vi "交换探头地址.vi"(8 "引用输入":T1, 11 "点到行列-实时列表":T2 caption="行和列") -> (2 "回滚成功？":bool, 3 "设置成功？":bool)   [LabVIEW 2017]
uses:
  <vilib>/Utility/miscctls.llb/LVRowAndColumnTypeDef.ctl
panel:
  out "引用-暂停发送":refnum<vi>
  in  "取消":bool
  in  "确定":bool
  in  "交换到探头":u8=1 min=1 max=35
  out "被修改探头":u8
  # "交换探头地址"
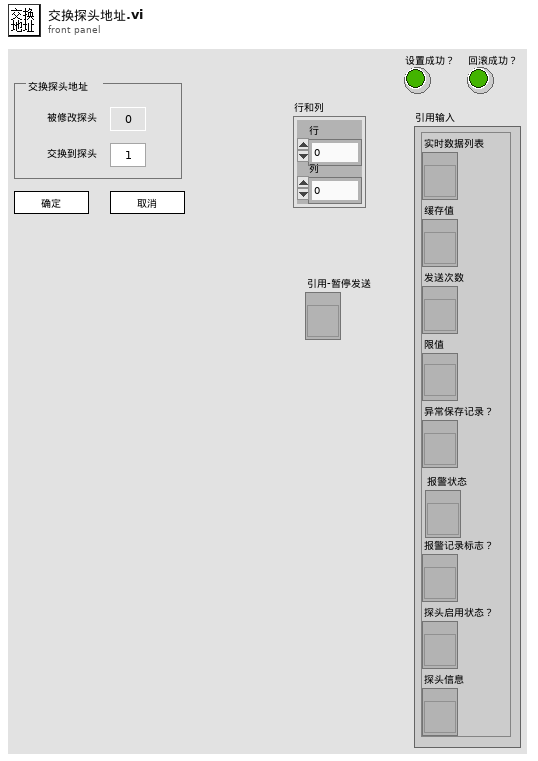
[diagram p1: front panel]
types:
  T1 = cluster{"实时数据列表":refnum<vi>, "缓存值":refnum<vi>, "发送次数":refnum<vi>, "限值":refnum<vi>, "异常保存记录？":refnum<vi>, "报警记录标志？":refnum<vi>, "探头启用状态？":refnum<vi>, "探头信息":refnum<vi>, "报警状态":refnum<vi>}
  T2 = typedef "LVRowAndColumnTypeDef.ctl" = cluster{"Row":i32, "Column":i32}
  T3 = enum32{"Invalid", "Standard", "Closed", "Hidden", "Minimized", "Maximized"}
  T4 = cluster{"限值1":dbl, "限值2":dbl, "探头限值":enum16{"一级限值", "二级限值"}}[]
  T5 = cluster{"限值1":dbl, "限值2":dbl, "探头限值":enum16{"一级限值", "二级限值"}}
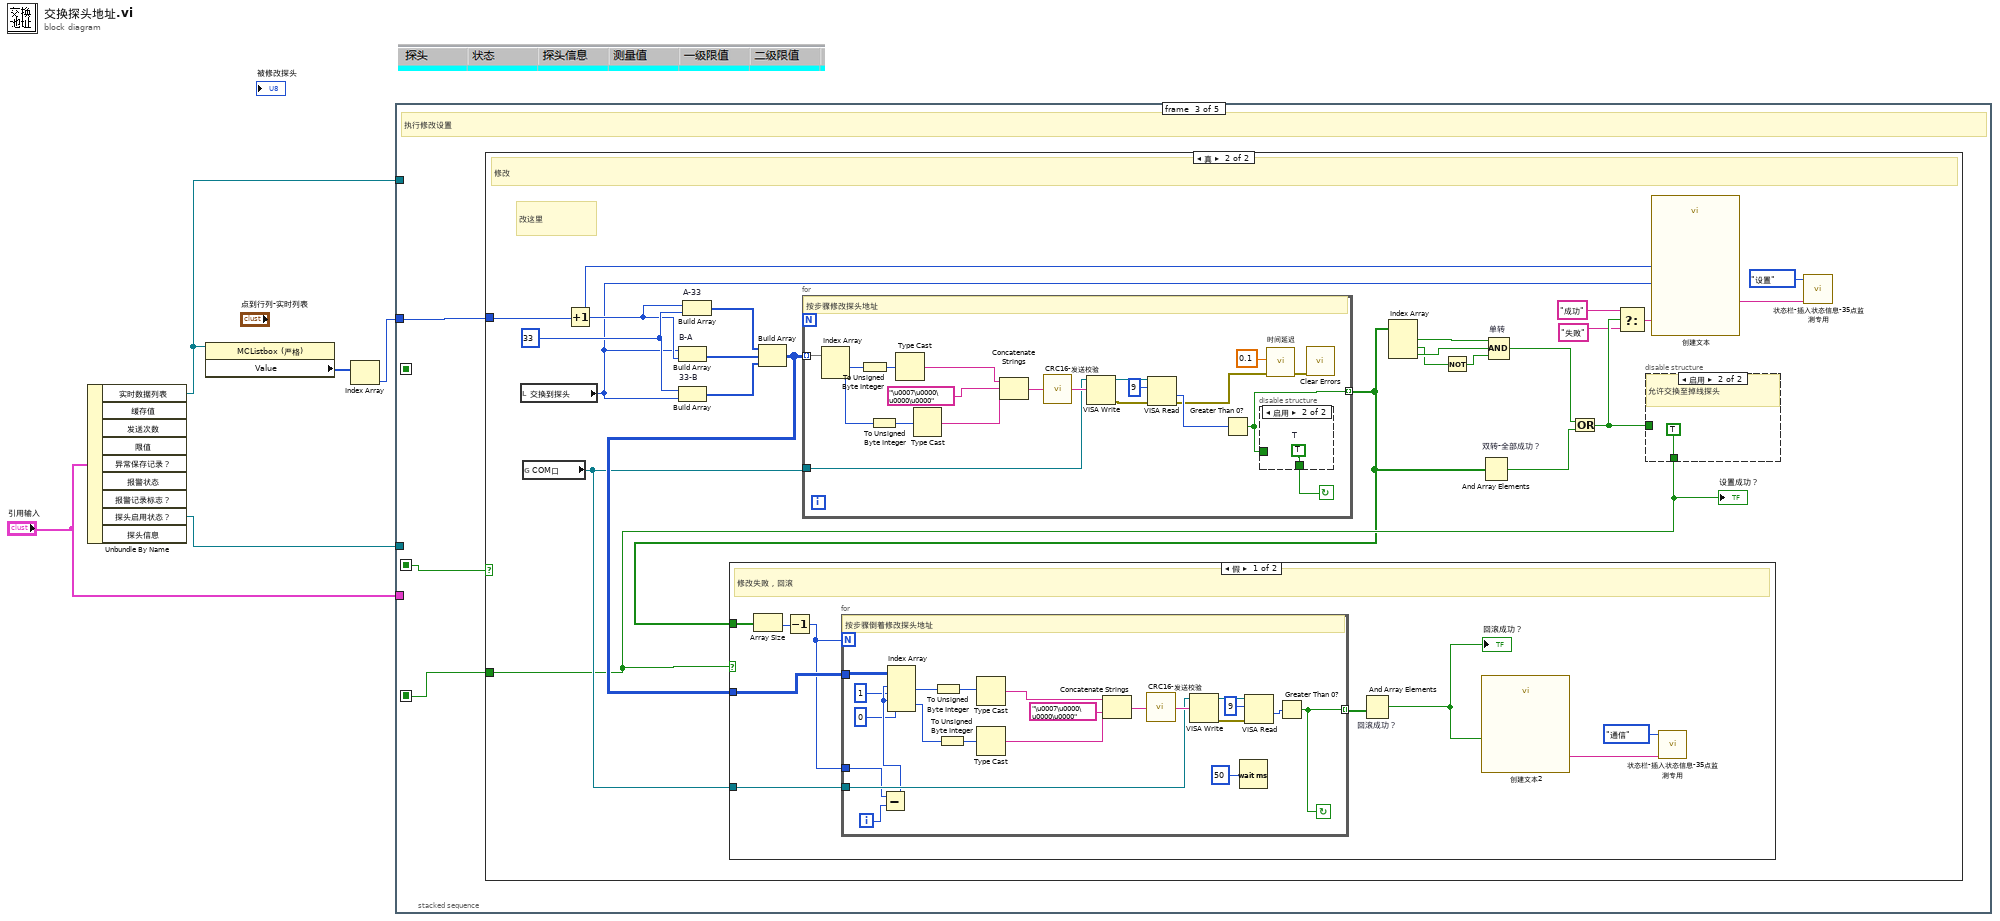
[diagram p0: block diagram]
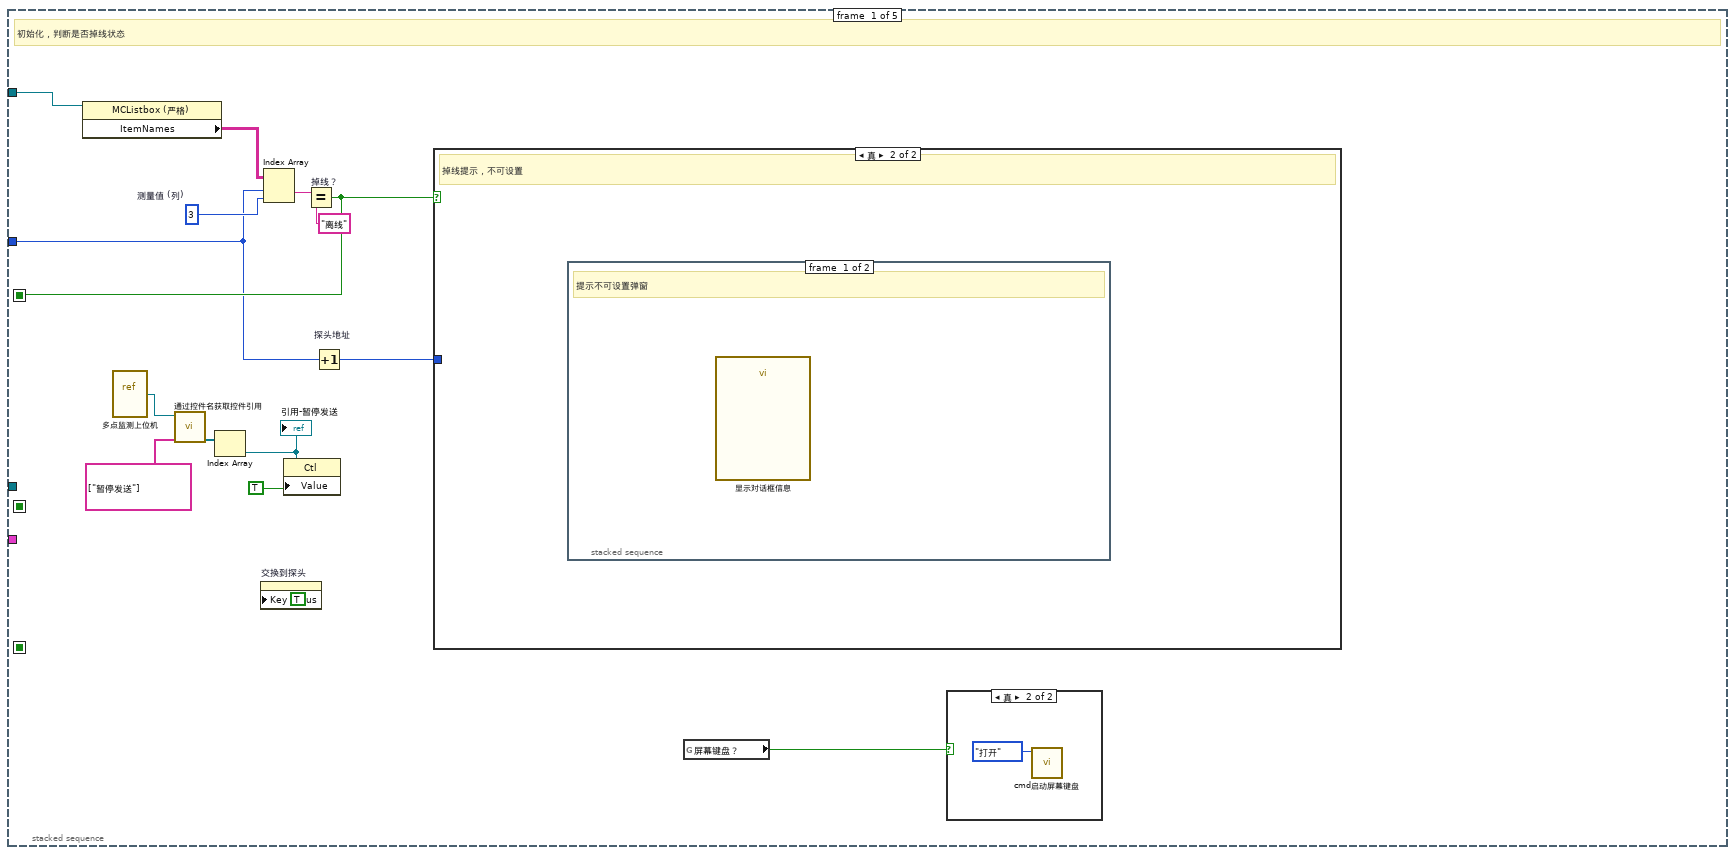
[diagram p2: hidden frame]
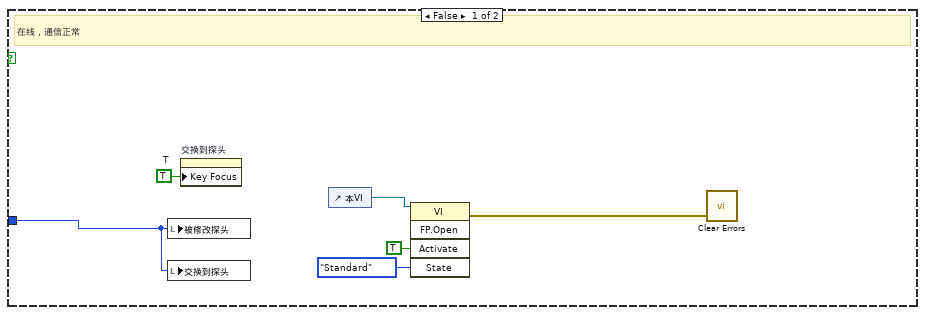
[diagram p4: hidden frame]
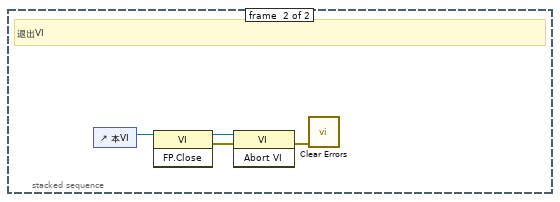
[diagram p5: hidden frame]
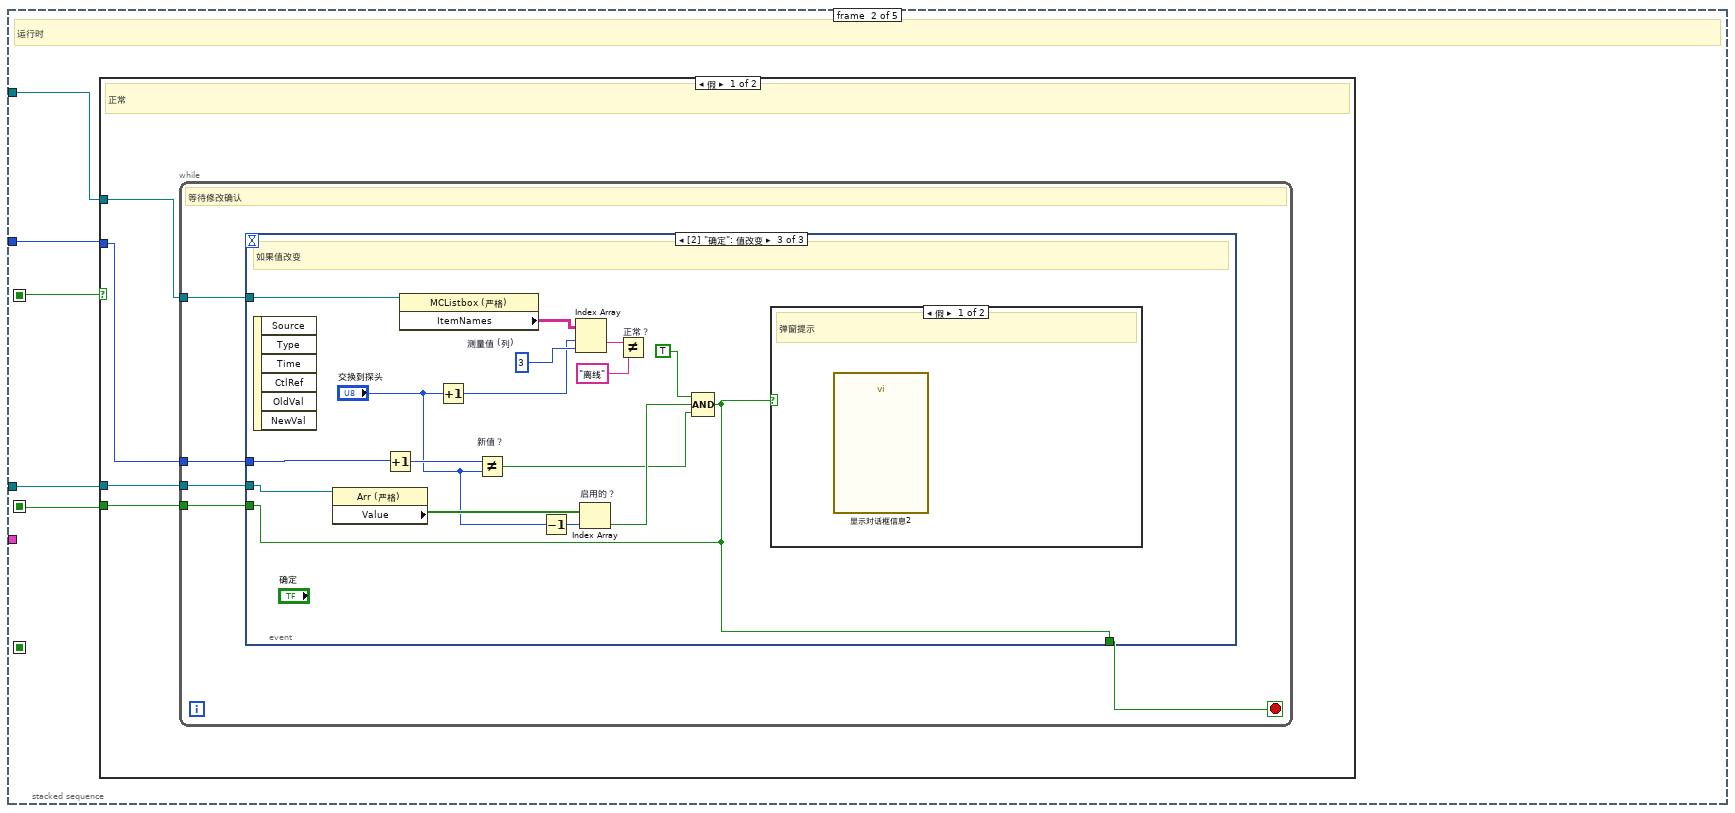
[diagram p6: hidden frame]
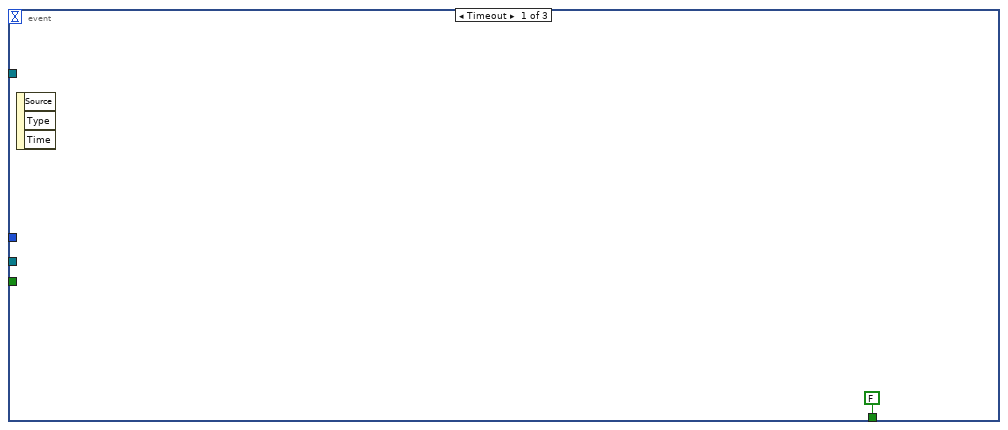
[diagram p7: hidden frame]
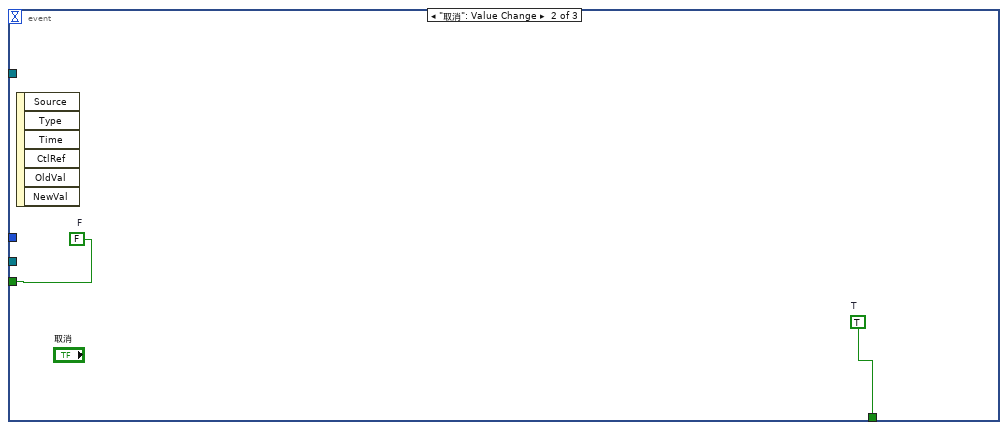
[diagram p8: hidden frame]
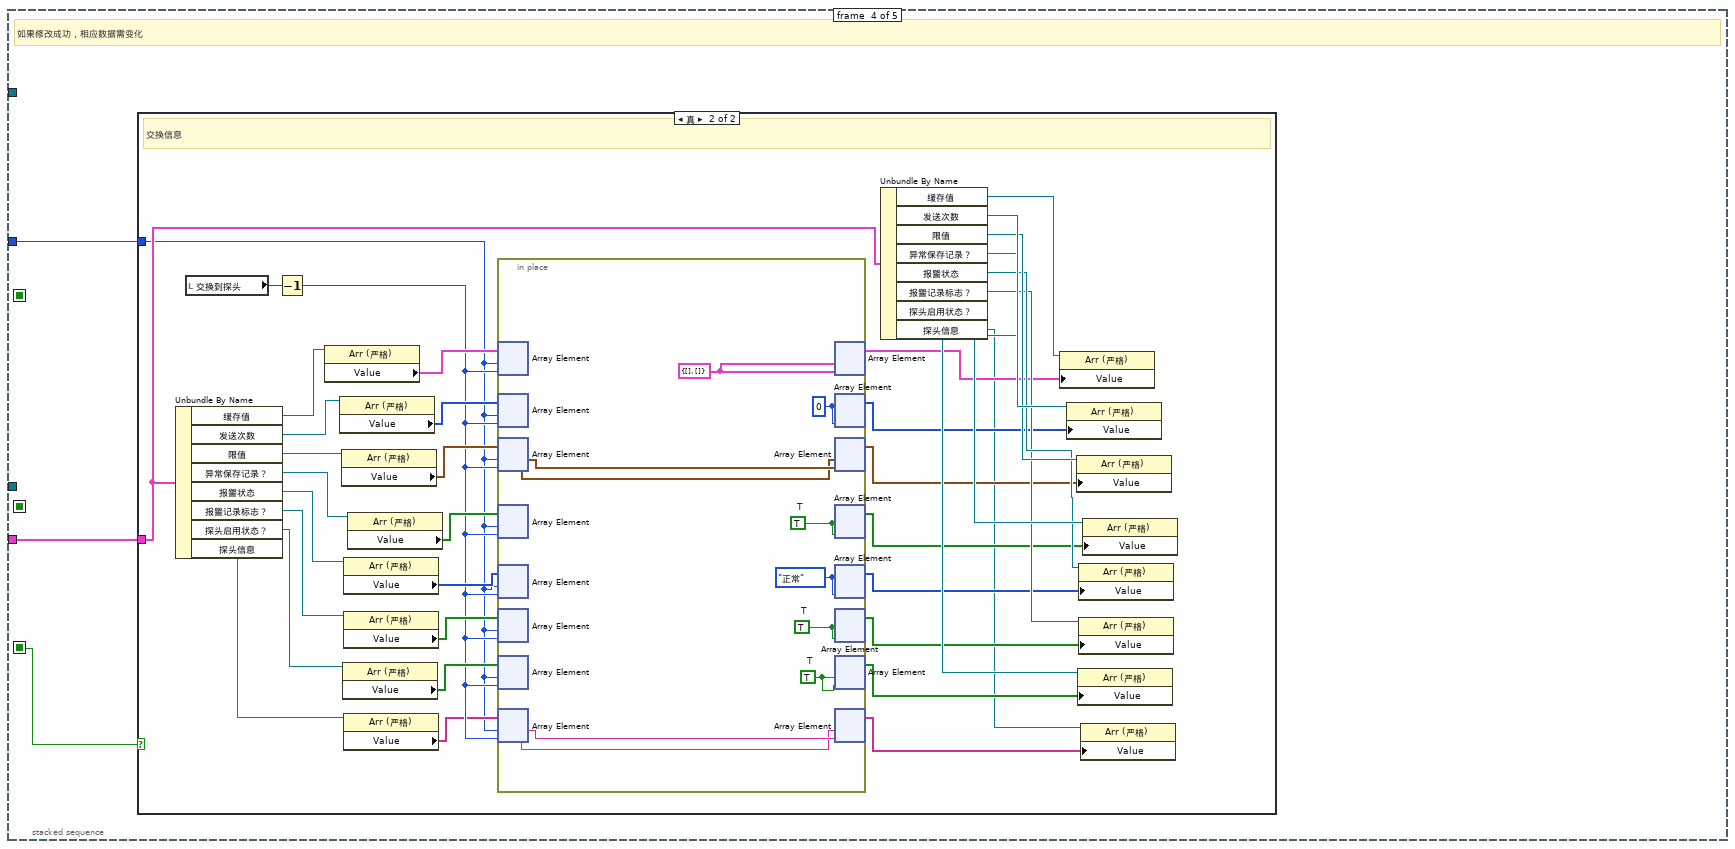
[diagram p15: hidden frame]
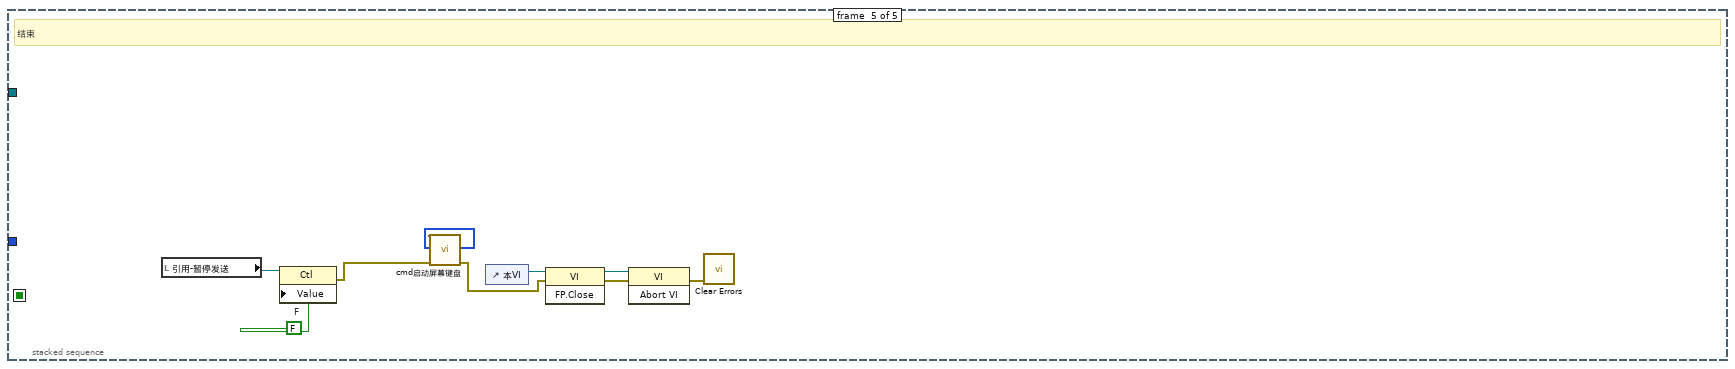
[diagram p17: hidden frame]
diagram:
  n1 = Unbundle By Name("引用输入") -> ("实时数据列表"=w3:refnum<vi>, "探头启用状态？"=w5:refnum<vi>)  [unwired: 7 out]
  n2 = property class="MCListbox (严格)"(reference=w3) -> ("Value"=w2:i32[])  [unwired: 1 in, 2 out]
  n3 = Index Array(array=w2) -> (element=w1:i32)  [unwired: 1 in]
  n4 = stacked-sequence {
    seq-local: [w15 _ _ _ _] -> [_ w36 _ _ _]
    seq-local: [_ w35 _ _ _] -> [_ _ w67 _ _]
    seq-local: [_ _ w66 _ _] -> [_ _ _ w148 _]
    tunnel: w3 -> [w20 w34 _ _ _]
    tunnel: w5 -> [_ w33 _ _ _]
    tunnel: "引用输入" -> [_ _ _ w147 _]
    tunnel: w1 -> [w13 w32 w65 w146 _]
    frame #0 {
      w18 = 3  # 测量值 (列)
      # "初始化，判断是否掉线状态"
      n5 = property class="MCListbox (严格)"(reference=w20) -> ("ItemNames"=w19:string[][])  [unwired: 1 in, 2 out]
      n6 = vi-ref "多点监测上位机.vi"() -> (w8:refnum<vi>)
      n7 = call "通过控件名获取控件引用.vi"("控件名数组"=string[] ["暂停发送"], "VI引用"=w8) -> ("控件引用输出"=w11:refnum<vi>[])  [unwired: 7 in, 2 out]
      n8 = Index Array(array=w11) -> (element=w9:refnum<vi>)  [unwired: 1 in]
      "引用-暂停发送" <- w9
      n9 = property on="交换到探头" class="DigNum (严格)"("Key Focus"=TRUE ("键选中")) -> ()  [unwired: 2 in, 2 out]
      n10 = Index Array(array=w19, index (row)=w13, index (col)=w18) -> (element=w17:string)
      n11 = property class="Ctl"(reference=w9, "Value"=TRUE ("T")) -> ()  [unwired: 1 in, 2 out]
      n12 = Equal? "掉线？"(x=w17, y="离线") -> (x = y?=w15:bool)
      n13 = Increment "探头地址"(x=w13) -> (x+1=w14:i32)
      n14 = case shown="真" w15 {
        tunnel: w14 -> [w27 _]
        frame False {
          w26 = TRUE  # T
          # "在线，通信正常"
          n15 = local write "被修改探头"(w27) -> ()
          n16 = local write "交换到探头"(w27) -> ()
          n17 = property on="交换到探头" class="DigNum (严格)"("Key Focus"=w26) -> ()  [unwired: 2 in, 2 out]
          n18 = control-ref of="本VI"() -> (w25:refnum<vi>)
          n19 = invoke class="VI" method="FP.Open"(reference=w25, "Activate"=TRUE ("激活？"), "State"=T3."Standard" ("状态")) -> (error out=w22:errorcluster)  [unwired: 2 in, 4 out]
          n20 = call <vilib>:"Clear Errors.vi"("error in (no error)"=w22) -> ()  [unwired: 5 in, 2 out]
        }
        frame True {
          # "掉线提示，不可设置"
          n21 = stacked-sequence {
            frame #0 {
              # "提示不可设置弹窗"
              n22 = call "显示对话框信息"() -> ()  [unwired: 10 in, 2 out]
            }
            frame #1 {
              # "退出VI"
              n23 = control-ref of="本VI"() -> (w31:refnum<vi>)
              n24 = invoke class="VI" method="FP.Close"(reference=w31) -> (reference out=w30:refnum<vi>, error out=w29:errorcluster)  [unwired: 2 in, 1 out]
              n25 = invoke class="VI" method="Abort VI"(reference=w30, error in=w29) -> (error out=w28:errorcluster)  [unwired: 1 in, 2 out]
              n26 = call <vilib>:"Clear Errors.vi"("error in (no error)"=w28) -> ()  [unwired: 5 in, 2 out]
            }
          }
        }
      }
      n27 = global read "全局变量-35点监测.vi" "屏幕键盘？"() -> (w6:bool)
      n28 = case shown="真" w6 {
        frame False {
        }
        frame True {
          n29 = call "cmd启动屏幕键盘.vi"("软键盘开关"=enum16{"关闭", "打开"}."打开") -> ()  [unwired: 9 in, 2 out]
        }
      }
    }
    frame #1 {
      # "运行时"
      n30 = case shown="假" w36 {
        tunnel: w32 -> [w39 _]
        tunnel: [w40 _] -> w35
        tunnel: w34 -> [w38 _]
        tunnel: w33 -> [w37 _]
        frame False {
          # "正常"
          n31 = while {
            tunnel: [w44] -> w40
            tunnel: w39 -> [w43]
            tunnel: w38 -> [w42]
            tunnel: w37 -> [w41]
            stop <- w45 stop-if-true
            # "等待修改确认"
            n32 = event shown="[2] \"确定\": 值改变" {
              selector: _ -> [_ _ _]
              dyn-events: _ -> [_ _ _]
              timeout: _ -> [_ _ _]
              tunnel: [FALSE ("T") w48 w54] -> w45
              tunnel: [_ w47 w54] -> w44
              tunnel: w43 -> [_ _ w53]
              tunnel: w42 -> [_ _ w59]
              tunnel: w41 -> [_ _ w58]
              event Timeout {
                n33 = event-data() -> ()  [unwired: 1 in, 3 out]
              }
              event "取消": Value Change {
                w47 = FALSE  # F
                w48 = TRUE  # T
                n34 = event-data() -> ()  [unwired: 1 in, 6 out]
              }
              event "确定": Value Change {
                w62 = 3  # 测量值 (列)
                # "如果值改变"
                n35 = event-data() -> ()  [unwired: 1 in, 6 out]
                n36 = property class="Arr (严格)"(reference=w58) -> ("Value"=w57:bool[])  [unwired: 1 in, 2 out]
                n37 = Increment(x=w53) -> (x+1=w64:i32)
                n38 = property class="MCListbox (严格)"(reference=w59) -> ("ItemNames"=w63:string[][])  [unwired: 1 in, 2 out]
                n39 = Increment(x="交换到探头") -> (x+1=w51:u8)
                n40 = Not Equal? "新值？"(x=w64, y="交换到探头") -> (x != y?=w55:bool)
                n41 = Decrement(x="交换到探头") -> (x-1=w49:u8)
                n42 = Index Array(array=w63, index (row)=w51, index (col)=w62) -> (element=w61:string)
                n43 = Index Array "启用的？"(array=w57, index=w49) -> (element=w56:bool)
                n44 = Not Equal? "正常？"(x=w61, y="离线") -> ()  [unwired: 1 out]
                n45 = Compound Arithmetic op=AND(TRUE ("值"), w56, w55) -> (w54:bool)
                n46 = case shown="假" w54 {
                  frame False {
                    # "弹窗提示"
                    n47 = call "显示对话框信息2"() -> ()  [unwired: 10 in, 2 out]
                  }
                  frame True {
                    # "正常，启用，新值"
                  }
                }
              }
            }
          }
        }
        frame True {
          # "掉线"
        }
      }
    }
    frame #2 {
      # "执行修改设置"
      n48 = case shown="真" w67 {
        tunnel: [_ w78] -> w66
        tunnel: w65 -> [_ w79]
        frame False {
          # "不执行"
        }
        frame True {
          w90 = 33 ("元素")
          # "改这里"
          # "修改"
          n49 = local read "交换到探头"() -> (w81:u8)
          n50 = global read "全局变量-35点监测.vi" "COM口"() -> (w84:refnum<visa-resource-name>)
          n51 = Increment(x=w79) -> (x+1=w82:i32)
          n52 = Build Array "B-A"(w81, w82) -> (w88:i32[])
          n53 = Build Array "33-B"(w90, w81) -> (w87:i32[])
          n54 = Build Array "A-33"(w82, w90) -> (w89:i32[])
          n55 = Build Array(w89, w88, w87) -> (w85:i32[][])
          n56 = for {
            tunnel: w85 -> [w143] mode=indexing
            tunnel: w84 -> [w131]
            tunnel: [w128] -> w73 mode=indexing
            stop <- w129 continue-if-true
            # "按步骤修改探头地址"
            n57 = Index Array(array=w143) -> (element #1=w137:i32, element #2=w136:i32)  [unwired: 2 in]
            n58 = To Unsigned Byte Integer(number=w137) -> (unsigned 8bit integer=w142:u8)
            n59 = To Unsigned Byte Integer(number=w136) -> (unsigned 8bit integer=w141:u8)
            n60 = Type Cast(x=w142) -> (*(type *) &x=w139:string)  [unwired: 1 in]
            n61 = Type Cast(x=w141) -> (*(type *) &x=w138:string)  [unwired: 1 in]
            n62 = Concatenate Strings(w139, "\u0007\u0000\u0000\u0000", w138) -> (w135:string)
            n63 = call "CRC16-发送校验.vi"("净数据"=w135) -> ("完整输出"=w132:string)
            n64 = VISA Write(VISA resource name=w131, write buffer=w132) -> (VISA resource name out=w134:refnum<visa-resource-name>, error out=w124:errorcluster)  [unwired: 1 in, 1 out]
            n65 = VISA Read(VISA resource name=w134, byte count=u32 9 ("字节总数"), error in (no error)=w124) -> (return count=w130:u32, error out=w127:errorcluster)  [unwired: 2 out]
            n66 = Greater Than 0?(x=w130) -> (x > 0?=w128:bool)
            n67 = disable-structure shown="启用" {
              disable-tunnel: [w144 w145] -> w129
              disable-tunnel: w128 -> [w144 _]
              frame Disabled {
              }
              frame Enabled {
                w145 = TRUE  # T
              }
            }
            n68 = call "时间延迟"("error in (no error)"=w127, "Delay Time (s)"=0.1) -> ("error out"=w126:errorcluster)  [unwired: 9 in]
            n69 = call <vilib>:"Clear Errors.vi"("error in (no error)"=w126) -> ()  [unwired: 5 in, 2 out]
          }
          n70 = Index Array(array=w73) -> (element #1=w72:bool, element #2=w70:bool, element #3=w71:bool)  [unwired: 3 in]
          n71 = Not(x=w70) -> (.not. x?=w69:bool)
          n72 = And Array Elements "双转-全部成功？"(Boolean array=w73) -> (logical AND=w86:bool)
          n73 = Compound Arithmetic op=AND "单转"(w72, w71, w69) -> (w68:bool)
          n74 = Or(x=w68, y=w86) -> (x .or. y?=w77:bool)
          n75 = Select(t="成功", s=w77, f="失败") -> (s? t:f=w74:string)
          n76 = disable-structure shown="启用" {
            disable-tunnel: w77 -> [w91 _]
            disable-tunnel: [w91 TRUE ("设置成功？")] -> w78
            frame Disabled {
              # "不允许交换至掉线探头"
            }
            frame Enabled {
              # "允许交换至掉线探头"
            }
          }
          "设置成功？" <- w78
          n77 = case shown="假" w78 {
            tunnel: w73 -> [w101 _]
            tunnel: w85 -> [w99 _]
            tunnel: w84 -> [w98 _]
            frame False {
              # "修改失败，回滚"
              n78 = Array Size(array=w101) -> (size(s)=w100:i32)
              n79 = Decrement(x=w100) -> (x-1=w97:i32)
              n80 = for {
                N: w97 -> [_]
                tunnel: w99 -> [w123]
                tunnel: w98 -> [w110]
                tunnel: [w107] -> w96 mode=indexing
                tunnel: w97 -> [w105]
                i -> [w106]
                stop <- w107 continue-if-true
                # "按步骤倒着修改探头地址"
                n81 = Subtract(x=w105, y=w106) -> (x-y=w104:i32)
                n82 = Index Array(array=w123, index (row) #1=w104, index (col) #1=1 ("禁用的索引 (列)"), index (row) #2=w104, index (col) #2=0 ("禁用的索引 (列)")) -> (element #1=w117:i32, element #2=w116:i32)
                n83 = To Unsigned Byte Integer(number=w117) -> (unsigned 8bit integer=w122:u8)
                n84 = To Unsigned Byte Integer(number=w116) -> (unsigned 8bit integer=w121:u8)
                n85 = Type Cast(x=w122) -> (*(type *) &x=w119:string)  [unwired: 1 in]
                n86 = Type Cast(x=w121) -> (*(type *) &x=w118:string)  [unwired: 1 in]
                n87 = Concatenate Strings(w119, "\u0007\u0000\u0000\u0000", w118) -> (w115:string)
                n88 = call "CRC16-发送校验.vi"("净数据"=w115) -> ("完整输出"=w111:string)
                n89 = VISA Write(VISA resource name=w110, write buffer=w111) -> (VISA resource name out=w113:refnum<visa-resource-name>, error out=w114:errorcluster)  [unwired: 1 in, 1 out]
                n90 = Wait (ms)(milliseconds to wait=u32 50 ("等待时间（毫秒）")) -> ()  [unwired: 1 out]
                n91 = VISA Read(VISA resource name=w113, byte count=u32 9 ("字节总数"), error in (no error)=w114) -> (return count=w108:u32)  [unwired: 3 out]
                n92 = Greater Than 0?(x=w108) -> (x > 0?=w107:bool)
              }
              n93 = And Array Elements "回滚成功？"(Boolean array=w96) -> (logical AND=w94:bool)
              "回滚成功？" <- w94
              n94 = call "创建文本2"("回滚成功？"=w94) -> ("Result"=w93:string)  [unwired: 13 in, 1 out]
              n95 = call "状态栏-插入状态信息-35点监测专用.vi"("消息内容"=w93, "状态类型"=enum16{"全部", "报警", "通信", "设置"}."通信") -> ()  [unwired: 10 in]
            }
            frame True {
              # "修改成功"
            }
          }
          n96 = call "创建文本"("从探头"=w82, "到探头"=w81, "交换结果"=w74) -> ("Result"=w80:string)  [unwired: 11 in, 1 out]
          n97 = call "状态栏-插入状态信息-35点监测专用.vi"("消息内容"=w80, "状态类型"=enum16{"全部", "报警", "通信", "设置"}."设置") -> ()  [unwired: 10 in]
        }
      }
    }
    frame #3 {
      # "如果修改成功，相应数据需变化"
      n98 = case shown="真" w148 {
        tunnel: w147 -> [_ w169]
        tunnel: w146 -> [_ w149]
        frame False {
        }
        frame True {
          # "交换信息"
          n99 = Unbundle By Name(w169) -> ("缓存值"=w183:refnum<vi>, "发送次数"=w181:refnum<vi>, "限值"=w179:refnum<vi>, "异常保存记录？"=w177:refnum<vi>, "报警状态"=w175:refnum<vi>, "报警记录标志？"=w173:refnum<vi>, "探头启用状态？"=w172:refnum<vi>, "探头信息"=w154:refnum<vi>)
          n100 = local read "交换到探头"() -> (w184:u8)
          n101 = Decrement(x=w184) -> (x-1=w153:u8)
          n102 = property class="Arr (严格)"(reference=w183) -> ("Value"=w182:cluster{"X":timestamp[], "Y":dbl[]}[])  [unwired: 1 in, 2 out]
          n103 = property class="Arr (严格)"(reference=w181) -> ("Value"=w180:u8[])  [unwired: 1 in, 2 out]
          n104 = property class="Arr (严格)"(reference=w179) -> ("Value"=w178:T4)  [unwired: 1 in, 2 out]
          n105 = property class="Arr (严格)"(reference=w172) -> ("Value"=w170:bool[])  [unwired: 1 in, 2 out]
          n106 = property class="Arr (严格)"(reference=w175) -> ("Value"=w174:enum16{"正常", "一级报警", "二级报警", "累积报警"}[])  [unwired: 1 in, 2 out]
          n107 = property class="Arr (严格)"(reference=w173) -> ("Value"=w171:bool[])  [unwired: 1 in, 2 out]
          n108 = property class="Arr (严格)"(reference=w154) -> ("Value"=w152:string[])  [unwired: 1 in, 2 out]
          n109 = property class="Arr (严格)"(reference=w177) -> ("Value"=w176:bool[])  [unwired: 1 in, 2 out]
          n110 = in-place {
            w187 = TRUE  # T
            w188 = TRUE  # T
            w189 = enum16{"正常", "一级报警", "二级报警"}."正常" ("元素")
            w190 = TRUE  # T
            w193 = u8 0 ("元素")
            w194 = cluster{"X":timestamp[], "Y":dbl[]} {"X"=[], "Y"=[]} ("元素")
            n111 = in-place-array #1(w182, w149, w153) -> ()  [unwired: 2 out]
            n112 = in-place-array #2(w180, w149, w153) -> ()  [unwired: 2 out]
            n113 = in-place-array #3(w178, w149, w153) -> (w192:T5, w191:T5)
            n114 = in-place-array #4(w176, w149, w153) -> ()  [unwired: 2 out]
            n115 = in-place-array #5(w174, w149, w153) -> ()  [unwired: 2 out]
            n116 = in-place-array #6(w171, w149, w153) -> ()  [unwired: 2 out]
            n117 = in-place-array #7(w170, w149, w153) -> ()  [unwired: 2 out]
            n118 = in-place-array #8(w152, w149, w153) -> (w186:string, w185:string)
            n119 = in-place-array #1(w194, w194) -> (w161:cluster{"X":timestamp[], "Y":dbl[]}[])  [unwired: 2 out]
            n120 = in-place-array #2(w193, w193) -> (w160:u8[])  [unwired: 2 out]
            n121 = in-place-array #3(w191, w192) -> (w159:T4)  [unwired: 2 out]
            n122 = in-place-array #4(w190, w190) -> (w158:bool[])  [unwired: 2 out]
            n123 = in-place-array #5(w189, w189) -> (w157:enum16{"正常", "一级报警", "二级报警", "累积报警"}[])  [unwired: 2 out]
            n124 = in-place-array #6(w188, w188) -> (w156:bool[])  [unwired: 2 out]
            n125 = in-place-array #7(w187, w187) -> (w155:bool[])  [unwired: 2 out]
            n126 = in-place-array #8(w185, w186) -> (w150:string[])  [unwired: 2 out]
          }
          n127 = Unbundle By Name(w169) -> ("缓存值"=w168:refnum<vi>, "发送次数"=w167:refnum<vi>, "限值"=w166:refnum<vi>, "异常保存记录？"=w165:refnum<vi>, "报警状态"=w164:refnum<vi>, "报警记录标志？"=w163:refnum<vi>, "探头启用状态？"=w162:refnum<vi>, "探头信息"=w151:refnum<vi>)
          n128 = property class="Arr (严格)"(reference=w168, "Value"=w161) -> ()  [unwired: 1 in, 2 out]
          n129 = property class="Arr (严格)"(reference=w167, "Value"=w160) -> ()  [unwired: 1 in, 2 out]
          n130 = property class="Arr (严格)"(reference=w166, "Value"=w159) -> ()  [unwired: 1 in, 2 out]
          n131 = property class="Arr (严格)"(reference=w162, "Value"=w155) -> ()  [unwired: 1 in, 2 out]
          n132 = property class="Arr (严格)"(reference=w164, "Value"=w157) -> ()  [unwired: 1 in, 2 out]
          n133 = property class="Arr (严格)"(reference=w163, "Value"=w156) -> ()  [unwired: 1 in, 2 out]
          n134 = property class="Arr (严格)"(reference=w151, "Value"=w150) -> ()  [unwired: 1 in, 2 out]
          n135 = property class="Arr (严格)"(reference=w165, "Value"=w158) -> ()  [unwired: 1 in, 2 out]
        }
      }
    }
    frame #4 {
      w199 = FALSE  # F
      # "结束"
      n136 = local read "引用-暂停发送"() -> (w198:refnum<vi>)
      n137 = property class="Ctl"(reference=w198, "Value"=w199) -> (error out=w196:errorcluster)  [unwired: 1 in, 1 out]
      n138 = call "cmd启动屏幕键盘.vi"("error in (no error)"=w196, "软键盘开关"=enum16{"关闭", "打开"}."关闭") -> ("error out"=w195:errorcluster)  [unwired: 8 in, 1 out]
      n139 = control-ref of="本VI"() -> (w203:refnum<vi>)
      n140 = invoke class="VI" method="FP.Close"(reference=w203, error in=w195) -> (reference out=w202:refnum<vi>, error out=w201:errorcluster)  [unwired: 1 in, 1 out]
      n141 = invoke class="VI" method="Abort VI"(reference=w202, error in=w201) -> (error out=w200:errorcluster)  [unwired: 1 in, 2 out]
      n142 = call <vilib>:"Clear Errors.vi"("error in (no error)"=w200) -> ()  [unwired: 5 in, 2 out]
    }
  }
